vi "PythonValue.vi"(6 "add self":bool=TRUE, 8 "error in":errorcluster, 11 "GObject in":refnum<class "GObject.lvclass">) -> (0 "error out":errorcluster, 3 "GObject out":refnum<class "GObject.lvclass">, 5 "value":string)   [LabVIEW 2014, in "Raspberry Pi Compatible Compiler for LabVIEW.lvlib" / "GObject.lvclass"]
uses:
  GObject.lvclass
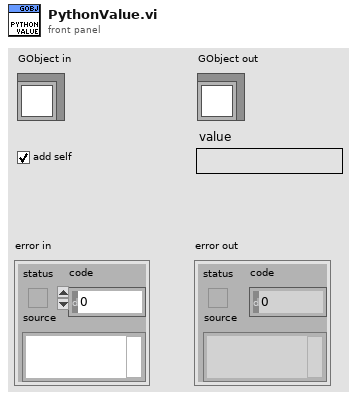
[diagram p1: front panel]
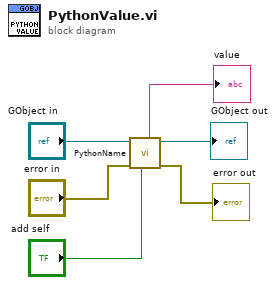
[diagram p0: block diagram]
diagram:
  n1 = call-dynamic "PythonName.vi"("add self"="add self", "error in"="error in", "GObject in"="GObject in") -> ("error out"=→"error out":errorcluster, "GObject out"=→"GObject out":refnum<class "GObject.lvclass">, "name"=→"value":string)  [unwired: 5 in, 1 out]
